vi "_r_n_HAPS.vi"() -> (2 "command":string)   [LabVIEW 2023, in "HAPS.lvlib"]
uses:
  HAPS.lvlib
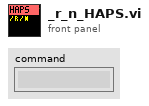
[diagram p1: front panel]
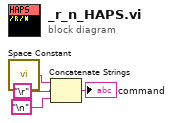
[diagram p0: block diagram]
diagram:
  n1 = call <vilib>:"Space Constant.vi"() -> ("String"=w4:string)
  n2 = Concatenate Strings(w4, "\r", "\n") -> (→"command":string)
